vi "Wakeup Helper Loop.vi"(8 "error in":errorcluster, 10 "HW ID":string) -> (0 "error out":errorcluster)   [LabVIEW 2024, in "Acquisition.lvlib"]
doc: "This is a private request to wake up the Helper Loop and start acquiring.\n_____\nCreated using DQMH Event Scripter 4.0.0.65.\n_____\nBased on DQMH Dev Tools: Project Template 7.1.0.1503."
uses:
  Acquisition.lvlib
  Wakeup Helper Loop Argument--cluster.ctl
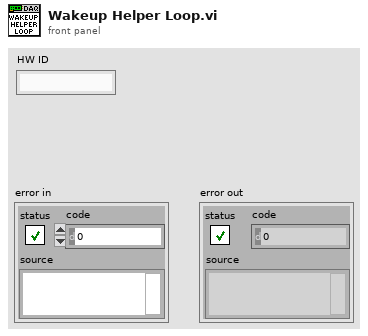
[diagram p1: front panel]
types:
  T1 = typedef "Acquisition.lvlib/Wakeup Helper Loop Argument--cluster.ctl" = cluster{"HW ID":string}
  T2 = typedef "Acquisition.lvlib/Request Events--cluster.ctl" = cluster{"Stop Module":refnum<user-event>, "Show Panel":refnum<user-event>, "Hide Panel":refnum<user-event>, "Get Module Execution Status":refnum<user-event>, "Show Diagram":refnum<user-event>, "Stop Acquiring":refnum<user-event>, "Wakeup Helper Loop":refnum<user-event>, "Change Settings":refnum<user-event>, "Calibrate DAQ":refnum<user-event>, "Start Acquiring":refnum<user-event>}
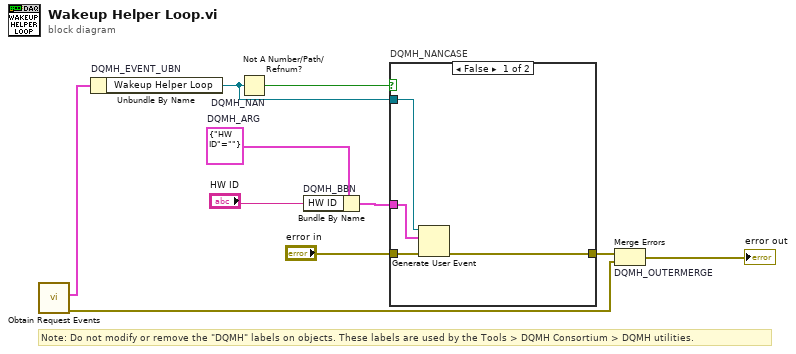
[diagram p0: block diagram]
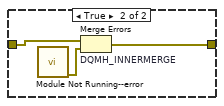
[diagram p2: hidden frame]
diagram:
  w4 = T1 {"HW ID"=""}  # DQMH_ARG
  # "Note: Do not modify or remove the \"DQMH\" labels on objects. These labels are used by the Tools > DQMH Consortium > DQMH utilities."
  n1 = call "Obtain Request Events.vi"() -> ("error out"=w3:errorcluster, "Acquisition Request Events"=w2:T2)  [unwired: 10 in]
  n2 = Unbundle By Name "DQMH_EVENT_UBN"(w2) -> ("Wakeup Helper Loop"=w6:refnum<user-event>)
  n3 = Not A Number/Path/Refnum? "DQMH_NAN"(number/path/refnum=w6) -> (NaN/Path/Refnum?=w7:bool)
  n4 = Bundle By Name "DQMH_BBN"(cluster=w4, "HW ID"="HW ID") -> (w8:T1)
  n5 = case "DQMH_NANCASE" shown="False" w7 {
    tunnel: "error in" -> [w14 w17]
    tunnel: [w13 w16] -> w5
    tunnel: w6 -> [w12 _]
    tunnel: w8 -> [w11 _]
    frame False {
      n6 = Generate User Event(user event=w12, event data cluster=w11, error in=w14) -> (error out=w13:errorcluster)  [unwired: 1 in, 1 out]
    }
    frame True {
      n7 = call "Module Not Running--error.vi"() -> ("error out"=w15:errorcluster)  [unwired: 11 in]
      n8 = Merge Errors "DQMH_INNERMERGE"(w17, w15) -> (w16:errorcluster)
    }
  }
  n9 = Merge Errors "DQMH_OUTERMERGE"(w5, w3) -> (→"error out":errorcluster)
